vi "init.vi"(0 "ROT Test in":refnum<class "ROT Test.lvclass">, 1 "Vref Channel To Read":refnum<k21>, 5 "Log":refnum<class "ITestLog.lvclass">, 7 "ILC Analog Output Test":T1 {"Tolerance" format="%.4f"; "Test Values"."Stop Value" format="%.6f"; "Test Values"."Start Value" format="%.6f"}, 9 "ILC":refnum<class "ILC.lvclass">, 11 "error in (no error)":errorcluster, 12 "Samples To Read":i32) -> (4 "ROT Test out":refnum<class "ROT Test.lvclass">, 15 "error out":errorcluster)   [LabVIEW 2015, in "ROT Test.lvclass"]
uses:
  ROT Test.lvclass
  <userlib>/Common/ILC/ILC/ILC.lvclass
  Typedefs/ILC Analog Output Test.ctl
  Typedefs/Test Values.ctl
  Model/TestLog/ITestLog/ITestLog.lvclass
  ROT Test.lvclass/ROT Test.ctl
  Typedefs/ILCBTTypedefs.lvlib
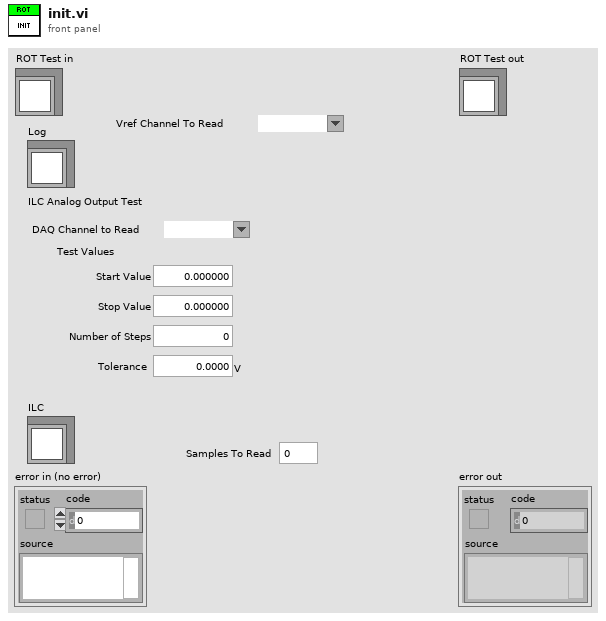
[diagram p1: front panel]
types:
  T1 = typedef "ILCBTTypedefs.lvlib/ILC Analog Output Test.ctl" = cluster{"DAQ Channel to Read":refnum<k21>, "Test Values":T2, "Tolerance":dbl[unit]}
  T2 = typedef "ILCBTTypedefs.lvlib/Test Values.ctl" = cluster{"Start Value":dbl, "Stop Value":dbl, "Number of Steps":u16}
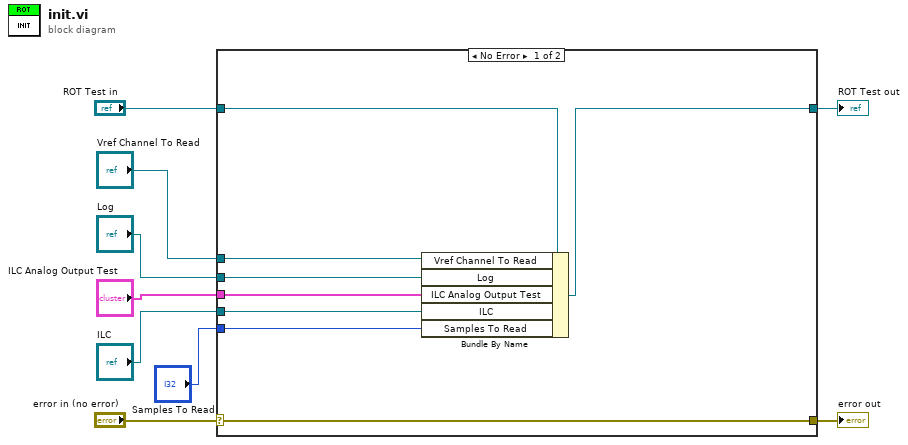
[diagram p0: block diagram]
diagram:
  n1 = case shown="No Error" "error in (no error)" {
    selector: "error in (no error)" -> [w17 w19]
    tunnel: [w17 w19] -> w8
    tunnel: [w15 w18] -> w6
    tunnel: "ROT Test in" -> [w16 w18]
    tunnel: "Log" -> [w14 _]
    tunnel: "ILC Analog Output Test" -> [w13 _]
    tunnel: "ILC" -> [w12 _]
    tunnel: "Vref Channel To Read" -> [w11 _]
    tunnel: "Samples To Read" -> [w10 _]
    frame No Error {
      n2 = Bundle By Name(cluster=w16, "Vref Channel To Read"=w11, "Log"=w14, "ILC Analog Output Test"=w13, "ILC"=w12, "Samples To Read"=w10) -> (w15:refnum<class "ROT Test.lvclass">)
    }
    frame Error {
    }
  }
  "error out" <- w8
  "ROT Test out" <- w6
